vi "Helper - Boolean to Log String.vi"(9 "Input":bool, 10 "Selector":string, 11 "PrevString":string) -> (3 "Output":string)   [LabVIEW 2011]
doc: "Part of Helper - Data to String.vi. Look there for more details."
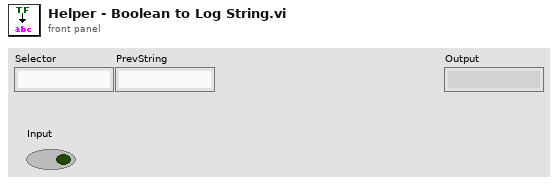
[diagram p1: front panel]
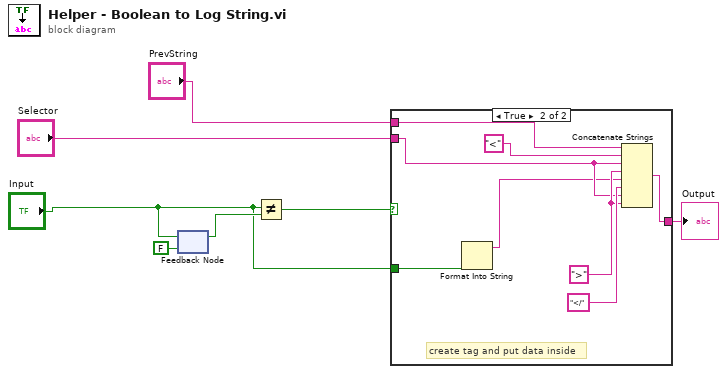
[diagram p0: block diagram]
diagram:
  n1 = feedback-in #1("Input") -> ()
  n2 = feedback #1(FALSE ("Input")) -> (w3:bool)
  n3 = Not Equal?(x="Input", y=w3) -> (x != y?=w4:bool)
  n4 = case shown="True" w4 {
    tunnel: [w8 w16] -> w6
    tunnel: "Selector" -> [_ w11]
    tunnel: "Input" -> [_ w10]
    tunnel: "PrevString" -> [w8 w12]
    frame False {
    }
    frame True {
      w13 = ">" ("string")
      # "create tag and put data inside"
      n5 = Format Into String(w10) -> (resulting string=w9:string)  [unwired: 3 in, 1 out]
      n6 = Concatenate Strings(w12, "<" ("string"), w11, w13, w9, "</" ("string"), w11, w13) -> (w16:string)
    }
  }
  "Output" <- w6
